vi "ExposeMapperGetType.vi"(10 "Value":variant, 11 "Data Val Ref in":refnum<data-value>) -> (0 "IsNumeric":bool, 1 "OType":T1=enum."Value", 2 "Name":string, 3 "DataType":T3, 4 "Container Type (Labview Value type)":T2, 5 "System Type":T4)   [LabVIEW 2017]
uses:
  <vilib>/Utility/Data Type/Type Definitions/Data Type.ctl
  ExposeMapperDataTypeEnum.ctl
  ExposeObjectMapContainerTypeEnum.ctl
  ExposeMapperObjectTypeEnum.ctl
  <vilib>/Utility/Data Type/NI_Data Type.lvlib
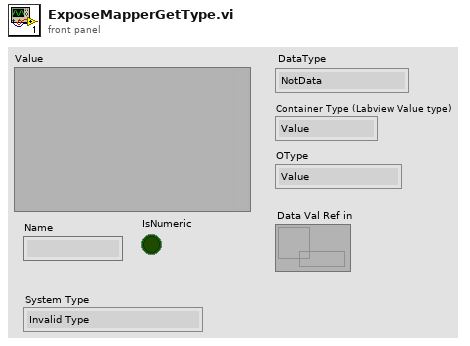
[diagram p1: front panel]
types:
  T1 = typedef "ExposeMapperObjectTypeEnum.ctl" = enum16{"NotAValidObject", "Value", "Variant", "Cluster", "Array", "Asng. Refnum"}
  T2 = typedef "ExposeObjectMapContainerTypeEnum.ctl" = enum16{"Value", "Array", "Waveform", "NetContainer"}
  T3 = typedef "ExposeMapperDataTypeEnum.ctl" = enum16{"NotData", "int8", "byte", "int16", "uint16", "int32", "uint32", "int64", "uint64", "Single", "Double", "String", "Boolean", "Container"}
  T4 = typedef "NI_Data Type.lvlib/Data Type.ctl" = enum8{"Invalid Type", "Void", "I8", "I16", "I32", "I64", "U8", "U16", "U32", "U64", "Single Float", "Double Float", "Extended Float", "Single Complex", "Double Complex", "Extended Complex", "Enum U8", "Enum U16", "Enum U32", "Enum U64", "Single Float With Unit", "Double Float With Unit", "Extended Float With Unit", "Single Complex with Unit", "Double Complex with Unit", "Extended Complex with Unit", "Boolean", "String", "Path", "Picture", "Tag", "Array", "Cluster", "Variant", "LV Variant", "Waveform", "Timestamp", "Digital Waveform", "Digital Data", "ExpressData", "Refnum", "External Data", "VI", "Poly VI", "LabVIEW Class Instance", "Fixed Point"}
  T5 = typedef "NI_Data Type.lvlib/Refnum Type.ctl" = enum16{"NotARefnum", "UnknownRefnum", "Generic", "Datalog", "ByteStream", "Device", "Occurence", "TCPNetConnection", "Auto", "Menu", "Imaq", "Hardware", "DataSocket", "Visa", "IVI", "UDPNetConnection", "Notifier", "Queue", "Irda", "EventReg", "DotNet", "UserEvent", "Callback", "UNUSED_EMPTY_POSITION", "BlueToothNetConnection", "LVObjApp", "LVObjVI", "LVObjUnknown", "GenericClass", "UserDefinedRefnumTag", "DataValue", "RT FIFO", "TDMS File"}
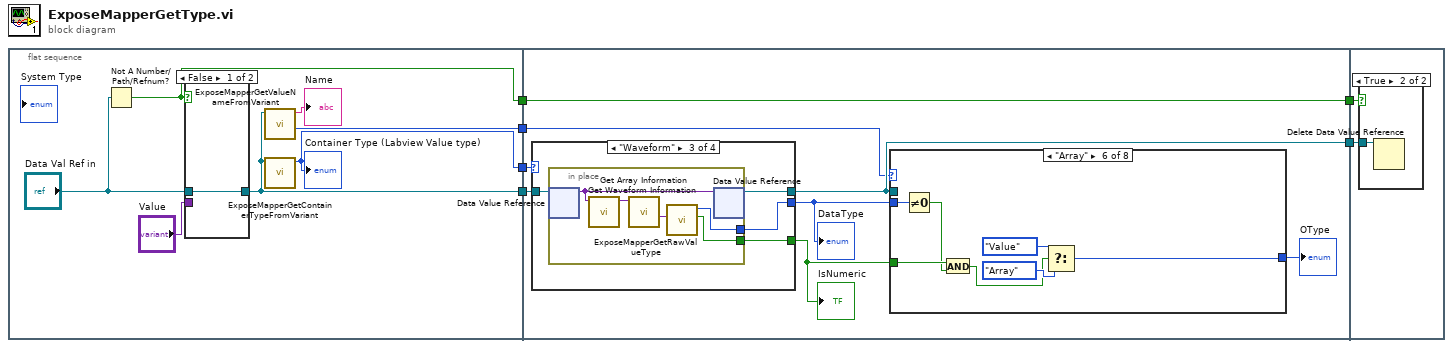
[diagram p0: block diagram]
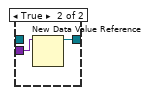
[diagram p2: hidden frame]
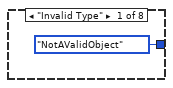
[diagram p3: hidden frame]
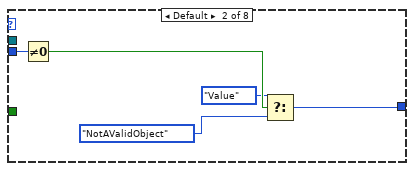
[diagram p4: hidden frame]
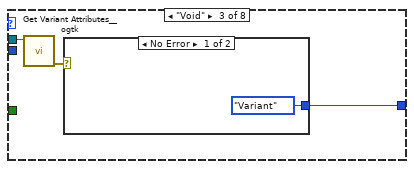
[diagram p5: hidden frame]
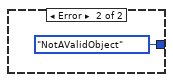
[diagram p6: hidden frame]
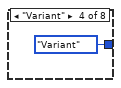
[diagram p7: hidden frame]
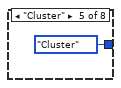
[diagram p8: hidden frame]
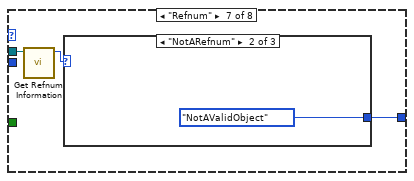
[diagram p9: hidden frame]
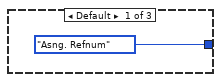
[diagram p10: hidden frame]
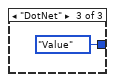
[diagram p11: hidden frame]
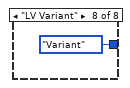
[diagram p12: hidden frame]
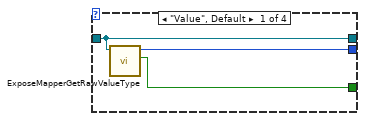
[diagram p13: hidden frame]
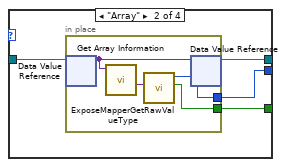
[diagram p14: hidden frame]
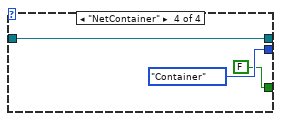
[diagram p15: hidden frame]
diagram:
  n1 = flat-sequence {
    tunnel: [w10] -> w4
    tunnel: [w9] -> w3
    tunnel: [w8] -> w2
    tunnel: [w7] -> w1
    tunnel: [w19] -> w6
    tunnel: [w21] -> w5
    tunnel: w4 -> [w20]
    tunnel: w3 -> [w19]
    tunnel: w2 -> [w18]
    tunnel: w1 -> [w17]
    tunnel: w6 -> [w76]
    tunnel: w5 -> [w75]
    frame #0 {
      n2 = Not A Number/Path/Refnum?(number/path/refnum="Data Val Ref in") -> (NaN/Path/Refnum?=w9:bool)
      n3 = case shown="False" w9 {
        tunnel: "Value" -> [_ w16]
        tunnel: [w14 w15] -> w10
        tunnel: "Data Val Ref in" -> [w14 _]
        frame False {
        }
        frame True {
          n4 = New Data Value Reference(data value=w16) -> (data value reference=w15:refnum<data-value>)  [unwired: 1 in, 1 out]
        }
      }
      n5 = call "ExposeMapperGetValueNameFromVariant.vi"("Data Val Ref in"=w10) -> ("System Type"=w7:T4, "Name"=→"Name":string)  [unwired: 9 in]
      n6 = call "ExposeMapperGetContainerTypeFromVariant.vi"("Data Val Ref in"=w10) -> ("LVPort Labview Contriner type"=w8:T2)  [unwired: 10 in]
      "Container Type (Labview Value type)" <- w8
    }
    frame #1 {
      n7 = case shown="\"Waveform\"" w18 {
        tunnel: w20 -> [w52 w56 w64 w72]
        tunnel: [w54 w58 w66 ExposeMapperDataTypeEnum."Container" ("MatlabType")] -> w24
        tunnel: [w53 w57 w65 FALSE ("IsNumeric")] -> w22
        tunnel: [w52 w55 w63 w72] -> w21
        frame "Value", Default {
          n8 = call "ExposeMapperGetRawValueType.vi"("Data Val Ref in"=w52) -> ("IsNumeric"=w53:bool, "MatlabType"=w54:T3)  [unwired: 9 in]
        }
        frame "Array" {
          n9 = in-place {
            in-place-border: [w62] -> w58
            in-place-border: [w61] -> w57
            n10 = in-place-dvr #1(w56) -> (w59:variant)  [unwired: 1 out]
            n11 = call <vilib>:"Get Array Information.vi"("Variant"=w59) -> ("Array Element Data Type"=w60:variant)  [unwired: 7 in, 3 out]
            n12 = call "ExposeMapperGetRawValueType.vi"("Value"=w60) -> ("IsNumeric"=w61:bool, "MatlabType"=w62:T3)  [unwired: 9 in]
            n13 = in-place-dvr #1(w59) -> (w55:refnum<data-value>)  [unwired: 1 out]
          }
        }
        frame "Waveform" {
          n14 = in-place {
            in-place-border: [w70] -> w66
            in-place-border: [w69] -> w65
            n15 = in-place-dvr #2(w64) -> (w68:variant)  [unwired: 1 out]
            n16 = call <vilib>:"Get Waveform Information.vi"("Variant"=w68) -> ("Y Array Type"=w71:variant)  [unwired: 9 in, 1 out]
            n17 = call <vilib>:"Get Array Information.vi"("Variant"=w71) -> ("Array Element Data Type"=w67:variant)  [unwired: 7 in, 3 out]
            n18 = call "ExposeMapperGetRawValueType.vi"("Value"=w67) -> ("IsNumeric"=w69:bool, "MatlabType"=w70:T3)  [unwired: 9 in]
            n19 = in-place-dvr #2(w68) -> (w63:refnum<data-value>)  [unwired: 1 out]
          }
        }
        frame "NetContainer" {
        }
      }
      "IsNumeric" <- w22
      "DataType" <- w24
      n20 = case shown="\"Array\"" w17 {
        tunnel: [ExposeMapperObjectTypeEnum."NotAValidObject" w27 w32 ExposeMapperObjectTypeEnum."Variant" ExposeMapperObjectTypeEnum."Cluster" w38 w47 ExposeMapperObjectTypeEnum."Variant"] -> w23
        tunnel: w24 -> [_ w26 _ _ _ w43 _ _]
        tunnel: w21 -> [_ _ w31 _ _ _ w46 _]
        tunnel: w22 -> [_ _ _ _ _ w41 _ _]
        frame "Invalid Type" {
        }
        frame Default {
          n21 = Not Equal To 0?(x=w26) -> (x != 0?=w30:bool)
          n22 = Select(t=ExposeMapperObjectTypeEnum."Value", s=w30, f=ExposeMapperObjectTypeEnum."NotAValidObject") -> (s? t:f=w27:T1)
        }
        frame "Void" {
          n23 = call <userlib>:"Get Variant Attributes__ogtk.vi"("Variant"=w31) -> ("error out"=w33:errorcluster)  [unwired: 3 in, 3 out]
          n24 = case shown="No Error" w33 {
            tunnel: [ExposeMapperObjectTypeEnum."Variant" ExposeMapperObjectTypeEnum."NotAValidObject"] -> w32
            frame No Error {
            }
            frame Error {
            }
          }
        }
        frame "Variant" {
        }
        frame "Cluster" {
        }
        frame "Array" {
          n25 = Not Equal To 0?(x=w43) -> (x != 0?=w40:bool)
          n26 = And(x=w41, y=w40) -> (x .and. y?=w39:bool)
          n27 = Select(t=ExposeMapperObjectTypeEnum."Value", s=w39, f=ExposeMapperObjectTypeEnum."Array") -> (s? t:f=w38:T1)
        }
        frame "Refnum" {
          n28 = call <vilib>:"Get Refnum Information.vi"("Variant"=w46) -> ("Reference Type"=w45:T5)  [unwired: 7 in, 3 out]
          n29 = case shown="\"NotARefnum\"" w45 {
            tunnel: [ExposeMapperObjectTypeEnum."Asng. Refnum" ("OType") ExposeMapperObjectTypeEnum."NotAValidObject" ExposeMapperObjectTypeEnum."Value"] -> w47
            frame Default {
            }
            frame "NotARefnum" {
            }
            frame "DotNet" {
            }
          }
        }
        frame "LV Variant" {
        }
      }
      "OType" <- w23
    }
    frame #2 {
      n30 = case shown="True" w76 {
        tunnel: w75 -> [_ w77]
        frame False {
        }
        frame True {
          n31 = Delete Data Value Reference(data value reference=w77) -> ()  [unwired: 1 in, 2 out]
        }
      }
    }
  }
